vi "Actor Core.vi"(8 "error in":errorcluster, 11 "Nested in":refnum<class "MXN Actor.lvclass">) -> (0 "error out":errorcluster, 3 "Actor out":refnum<class "Actor.lvclass">)   [LabVIEW 2019, in "MXN Actor.lvlib" / "MXN Actor.lvclass"]
doc: "(<B>Filename</B>: Actor Framework.lvlib:Actor.lvclass:Actor Core.vi)\n\nReceives messages to the actor, reacts to them, and initiates any error handling that may shut the actor down.\n\nDescendant classes may override this VI to append parallel tasks for the actor to complete while it handles messages. Overrides use the Call Parent Method node."
uses:
  MXN Actor.lvclass
  C:/Program Files/National Instruments/LabVIEW 2019/vi.lib/ActorFramework/Actor/Actor.lvclass
  <vilib>/ActorFramework/Actor/Actor.lvclass
  <vilib>/ActorFramework/Actor/Actor.lvclass/Actor.ctl
  <vilib>/ActorFramework/Message Enqueuer/Message Enqueuer.lvclass/Message Enqueuer.ctl
  MXN Actor.lvclass/MXN Actor.ctl
  MXN Actor Messages/Process coin Msg/Process coin Msg.lvclass/Process coin Msg.ctl
  <vilib>/ActorFramework/Message Enqueuer/Init from Existing Queue.vi
  <vilib>/ActorFramework/Message Enqueuer/Enqueue.vi
  <vilib>/Utility/error.llb/Clear Errors.vi
  <vilib>/ActorFramework/Stop Msg/Stop Msg.lvclass
  C:/Program Files/National Instruments/LabVIEW 2019/vi.lib/ActorFramework/Message/Message.lvclass
  MXN Actor Messages/Process coin Msg/Process coin Msg.lvclass
  <vilib>/ActorFramework/Message Priority Queue/Priority Enqueue.vi
  <vilib>/ActorFramework/Message Enqueuer/Message Enqueuer.lvclass
panel:
  in  "Coins":T1
  # "MXN"
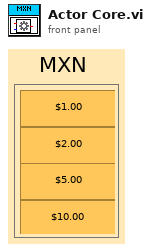
[diagram p1: front panel]
types:
  T1 = cluster{"1":bool, "1 2":bool, "1 3":bool, "1 4":bool}
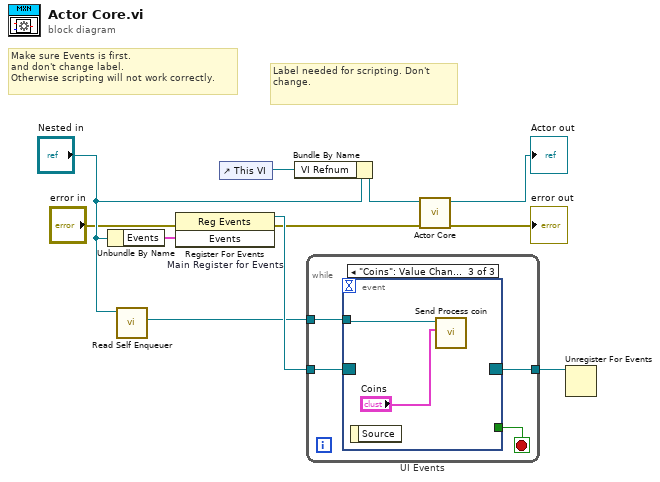
[diagram p0: block diagram]
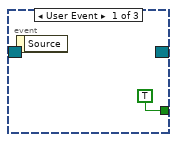
[diagram p2: hidden frame]
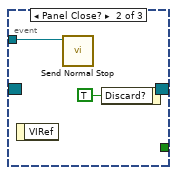
[diagram p3: hidden frame]
diagram:
  # "Label needed for scripting. Don't change."
  # "Make sure Events is first.\nand don't change label.\nOtherwise scripting will not work correctly."
  n1 = Unbundle By Name("Nested in") -> ("Events"=w8:cluster{"Stop":refnum<user-event>})
  n2 = call <vilib>:"Read Self Enqueuer.vi"("Actor"="Nested in") -> ("Self Enqueuer"=w5:refnum<class "Message Enqueuer.lvclass">)  [unwired: 10 in]
  n3 = register-events "Main Register for Events"(error in="error in", w8) -> (reference out=w9:refnum<event-registration>, error out=w3:errorcluster)  [unwired: 1 in]
  n4 = control-ref of="This VI"() -> (w1:refnum<vi>)
  n5 = Bundle By Name(cluster="Nested in", "VI Refnum"=w1) -> (w2:refnum<class "MXN Actor.lvclass">)
  n6 = while {
    tunnel: w9 -> [w15]
    tunnel: [w13] -> w7
    tunnel: w5 -> [w12]
    stop <- w14 stop-if-true
    n7 = event "UI Events" shown="[2] \"Coins\": Value Change" {
      selector: w15 -> [_ _ _]
      dyn-events: [_ _ _] -> w13
      timeout: _ -> [_ _ _]
      tunnel: [TRUE _ _] -> w14
      tunnel: w12 -> [_ w17 w20]
      event User Event {
        n8 = event-data() -> ()  [unwired: 1 in, 1 out]
      }
      event Panel Close? {
        n9 = event-data() -> ()  [unwired: 1 in, 1 out]
        n10 = call <vilib>:"Send Normal Stop.vi"("Message Enqueuer"=w17) -> ()  [unwired: 10 in, 1 out]
        n11 = event-data("Discard?"=TRUE) -> ()  [unwired: 1 in, 1 out]
      }
      event "Coins": Value Change {
        n12 = event-data() -> ()  [unwired: 1 in, 1 out]
        n13 = call "Send Process coin.vi"("Coins"="Coins", "Message Enqueuer"=w20) -> ()  [unwired: 8 in, 2 out]
      }
    }
  }
  n14 = call-parent "Actor Core.vi"("error in"=w3, "Actor in"=w2) -> ("error out"=→"error out":errorcluster, "Actor out"=→"Actor out":refnum<class "Actor.lvclass">)  [unwired: 8 in]
  n15 = Unregister For Events(event registration refnum=w7) -> ()  [unwired: 1 in, 1 out]
